vi "FGV Status Lambda.vi"(6 "Aktionen":T2, 8 "error in":errorcluster caption="Fehler", 11 "Istwerte":sgl[](array[numeric])) -> (2 "Lambda Fehler":T1, 3 "Istwerte":sgl[](array[numeric]))   [LabVIEW 2020, in "Lambda_ Komm.lvlib"]
uses:
  Lambda_ Komm.lvlib
  FGV Status Lambda Aktionen.ctl
  Lambda Fehler.ctl
panel:
  # "Lambda\nRi\nO2\nA/F"
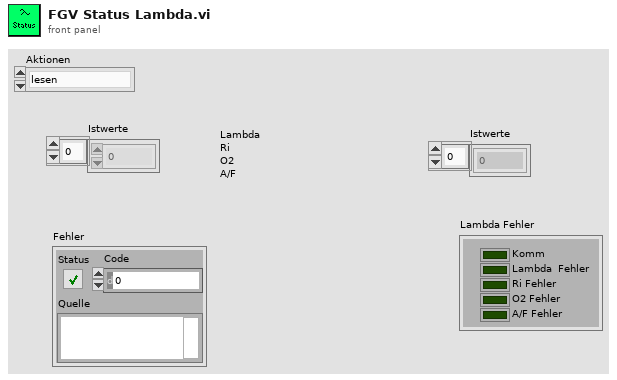
[diagram p1: front panel]
types:
  T1 = typedef "Lambda_ Komm.lvlib/Lambda Fehler.ctl" = cluster{"Komm":bool, "Lambda  Fehler":bool, "Ri Fehler":bool, "O2 Fehler":bool, "A/F Fehler":bool}
  T2 = typedef "Lambda_ Komm.lvlib/FGV Status Lambda Aktionen.ctl" = enum16{"lesen", "init", "Istwerte"}
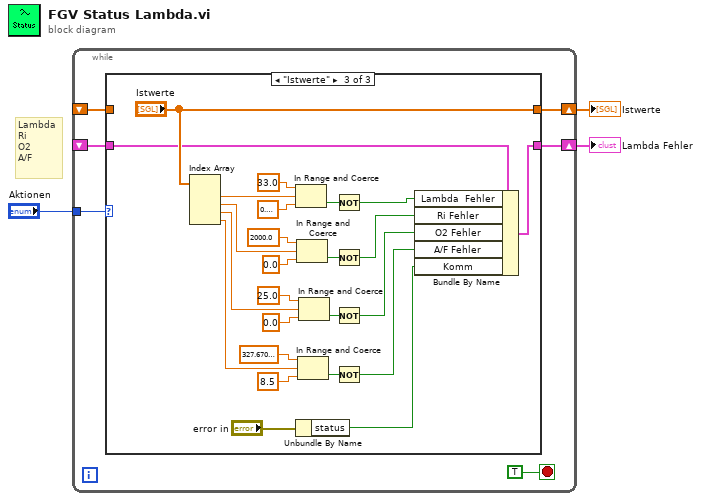
[diagram p0: block diagram]
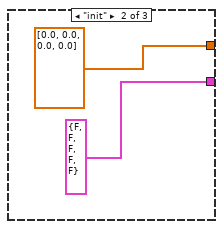
[diagram p3: hidden frame]
diagram:
  # "Lambda\nRi\nO2\nA/F"
  n1 = while {
    tunnel: "Aktionen" -> [w8]
    shift-right: [w7] -> w2
    shift-left: _ -> [w6]
    shift-right: [w4] -> w1
    shift-left: _ -> [w5]
    stop <- TRUE stop-if-true
    n2 = case shown="\"Istwerte\"" w8 {
      tunnel: [w11 sgl[] [0.0, 0.0, 0.0, 0.0] ("Istwerte") "Istwerte"] -> w7
      tunnel: w6 -> [w11 _ _]
      tunnel: w5 -> [w10 _ w21]
      tunnel: [w10 T1 {"Komm"=FALSE, "Lambda  Fehler"=FALSE, "Ri Fehler"=FALSE, "O2 Fehler"=FALSE, "A/F Fehler"=FALSE} ("Lambda Fehler") w20] -> w4
      frame "lesen", Default {
      }
      frame "init" {
      }
      frame "Istwerte" {
        n3 = Index Array(array="Istwerte") -> (element #1=w37:sgl, element #2=w28:sgl, element #3=w27:sgl, element #4=w26:sgl)  [unwired: 4 in]
        n4 = In Range and Coerce(upper limit=sgl 33.0 ("Obergrenze"), x=w37, lower limit=sgl 0.6 ("Untergrenze")) -> (In Range?=w25:bool)  [unwired: 1 out]
        n5 = Unbundle By Name("error in") -> ("status"=w14:bool)
        n6 = In Range and Coerce(upper limit=sgl 2000.0 ("Obergrenze"), x=w28, lower limit=sgl 0.0 ("Untergrenze")) -> (In Range?=w22:bool)  [unwired: 1 out]
        n7 = In Range and Coerce(upper limit=sgl 327.67 ("Obergrenze"), x=w26, lower limit=sgl 8.5 ("Untergrenze")) -> (In Range?=w24:bool)  [unwired: 1 out]
        n8 = In Range and Coerce(upper limit=sgl 25.0 ("Obergrenze"), x=w27, lower limit=sgl 0.0 ("Untergrenze")) -> (In Range?=w23:bool)  [unwired: 1 out]
        n9 = Not(x=w25) -> (.not. x?=w16:bool)
        n10 = Not(x=w22) -> (.not. x?=w19:bool)
        n11 = Not(x=w23) -> (.not. x?=w18:bool)
        n12 = Not(x=w24) -> (.not. x?=w17:bool)
        n13 = Bundle By Name(cluster=w21, "Lambda  Fehler"=w16, "Ri Fehler"=w19, "O2 Fehler"=w18, "A/F Fehler"=w17, "Komm"=w14) -> (w20:T1)
      }
    }
  }
  "Istwerte" <- w2
  "Lambda Fehler" <- w1
